vi "AddEntry2Table.vi"(6 "Dwell Time @ SP (sec)":u32 step=1 format="%.0f sec", 8 "error in (no error)":errorcluster, 9 "Cooling rate (°C/min)":dbl=0.01 min=0.01 max=5.0 step=0.01 format="%.2g °C/min", 10 "SP (°C)":dbl min=-50.0 max=50.0 step=0.1 format="%.1g °C", 11 "RampProgramModel in":refnum<class "RampProgramModel.lvclass">) -> (0 "error out":errorcluster, 3 "RampProgramModel out":refnum<class "RampProgramModel.lvclass">)   [LabVIEW 2013, in "RampProgramModel.lvclass"]
uses:
  RampProgramModel.lvclass
  RampProgramModel.lvclass/RampProgramModel.ctl
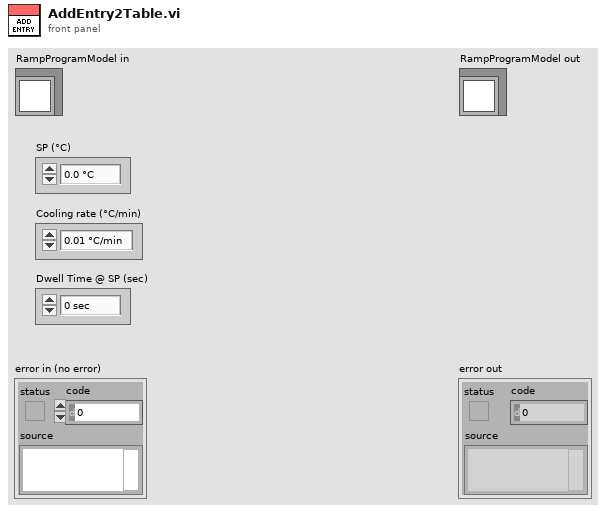
[diagram p1: front panel]
types:
  T1 = cluster{"SP (°C)":dbl, "Cooling rate (°C/min)":dbl, "Dwell Time @ SP (sec)":u32}
  T2 = cluster{"SP (°C)":dbl, "Cooling rate (°C/min)":dbl, "Dwell Time @ SP (sec)":u32}[]
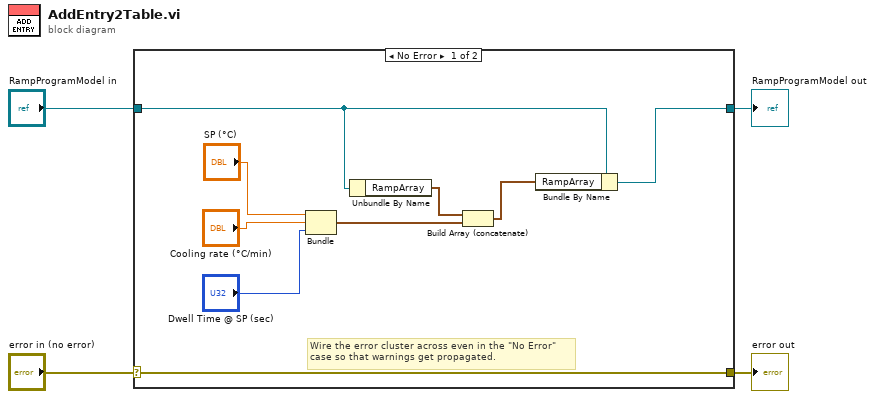
[diagram p0: block diagram]
diagram:
  n1 = case shown="No Error" "error in (no error)" {
    selector: "error in (no error)" -> [w13 w15]
    tunnel: [w13 w15] -> w3
    tunnel: [w12 w14] -> w1
    tunnel: "RampProgramModel in" -> [w7 w14]
    frame No Error {
      # "Wire the error cluster across even in the \"No Error\"\ncase so that warnings get propagated."
      n2 = Bundle("SP (°C)"="SP (°C)", "Cooling rate (°C/min)"="Cooling rate (°C/min)", "Dwell Time @ SP (sec)"="Dwell Time @ SP (sec)") -> (w8:T1)  [unwired: 1 in]
      n3 = Unbundle By Name(w7) -> ("RampArray"=w6:T2)
      n4 = Build Array (concatenate)(w6, w8) -> (w5:T2)
      n5 = Bundle By Name(cluster=w7, "RampArray"=w5) -> (w12:refnum<class "RampProgramModel.lvclass">)
    }
    frame Error {
    }
  }
  "error out" <- w3
  "RampProgramModel out" <- w1
